vi "Get Category.vi"(8 "error in (no error)":errorcluster, 11 "ScaleAndLimitModule editor node in":refnum<class "ScaleAndLimitModule editor node.lvclass">) -> (0 "error out":errorcluster, 2 "Category":string, 3 "ScaleAndLimitModule editor node out":refnum<class "ScaleAndLimitModule editor node.lvclass">)   [LabVIEW 2017, in "ScaleAndLimitModule editor node.lvclass"]
uses:
  ScaleAndLimitModule editor node.lvclass
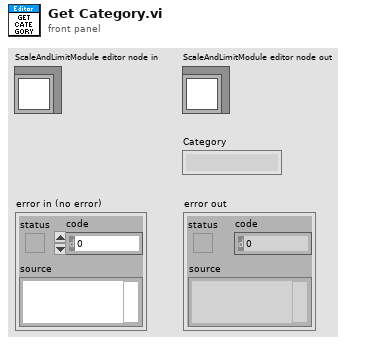
[diagram p1: front panel]
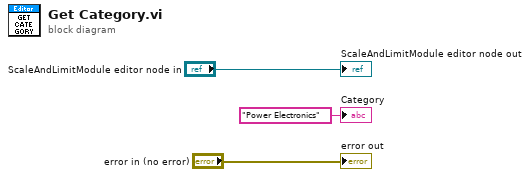
[diagram p0: block diagram]
diagram:
  "error out" <- "error in (no error)"
  "ScaleAndLimitModule editor node out" <- "ScaleAndLimitModule editor node in"
  "Category" <- "Power Electronics" ("Category")
